vi "Update-motor-status.vi"(8 "error in (no error)":errorcluster, 11 "Object ref in":T1) -> (0 "error out":errorcluster, 3 "Object ref out":T1)   [LabVIEW 2013, in "PowderDeposition.lvlib" / "PD-Main.lvclass"]
uses:
  PD-Main.lvclass
  Object-reference.ctl
  PD-Main.lvclass/PD-Main.ctl
  Assembly/Motor-assembly.lvclass
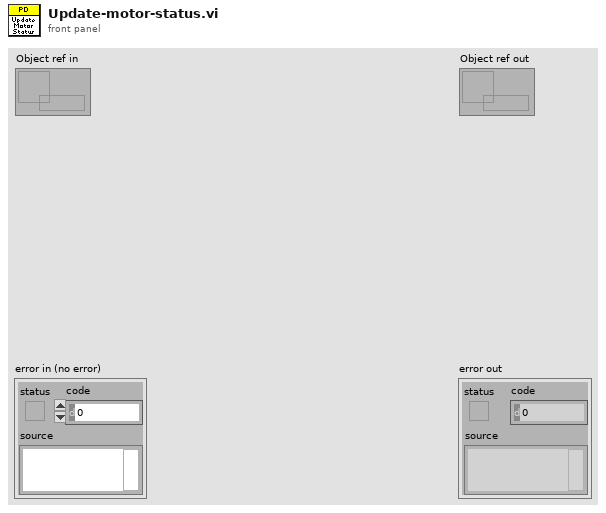
[diagram p1: front panel]
types:
  T1 = typedef "PowderDeposition.lvlib/PD-Main.lvclass/Object-reference.ctl" = refnum<data-value>
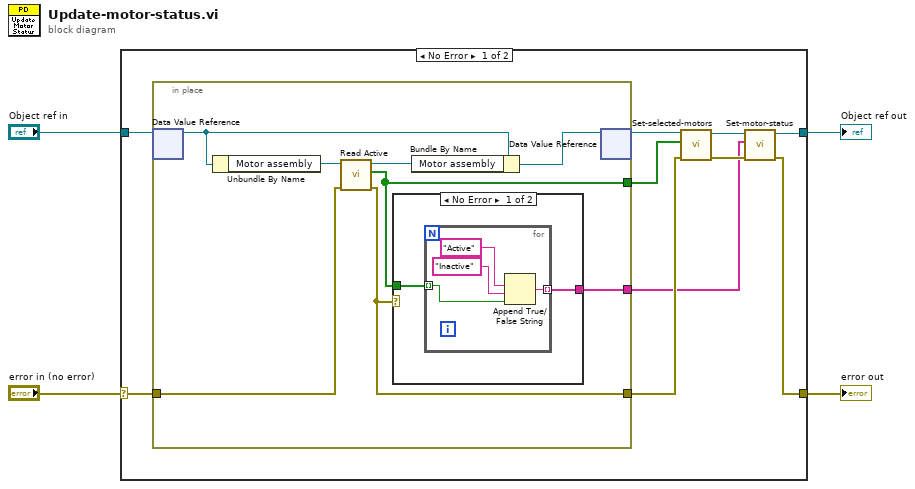
[diagram p0: block diagram]
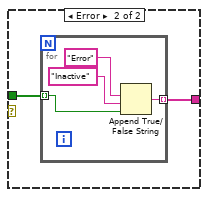
[diagram p2: hidden frame]
diagram:
  n1 = case shown="No Error" "error in (no error)" {
    selector: "error in (no error)" -> [w13 w36]
    tunnel: [w9 w36] -> w3
    tunnel: [w10 w35] -> w1
    tunnel: "Object ref in" -> [w14 w35]
    frame No Error {
      n2 = in-place {
        in-place-border: [w21] -> w8
        in-place-border: w13 -> [w20]
        in-place-border: [w16] -> w5
        in-place-border: [w15] -> w6
        n3 = in-place-dvr #1(w14) -> (w18:refnum<class "PD-Main.lvclass">)  [unwired: 1 out]
        n4 = Unbundle By Name(w18) -> ("Motor assembly"=w22:refnum<class "Motor-assembly.lvclass">)
        n5 = call-dynamic "Read Active.vi"("error in (no error)"=w20, "Available motors in"=w22) -> ("error out"=w21:errorcluster, "Active?"=w15:bool[], "Available motors out"=w19:refnum<class "Motor-assembly.lvclass">)  [unwired: 7 in]
        n6 = case shown="No Error" w21 {
          tunnel: w15 -> [w23 w30]
          tunnel: [w24 w29] -> w16
          frame No Error {
            n7 = for {
              tunnel: w23 -> [w28] mode=indexing
              tunnel: [w25] -> w24 mode=indexing
              n8 = Append True/False String(1:w28, 2:"Inactive" ("true string"), 3:"Active" ("true string")) -> (0:w25:string)  [unwired: 1 in]
            }
          }
          frame Error {
            n9 = for {
              tunnel: w30 -> [w34] mode=indexing
              tunnel: [w31] -> w29 mode=indexing
              n10 = Append True/False String(1:w34, 2:"Inactive" ("true string"), 3:"Error" ("true string")) -> (0:w31:string)  [unwired: 1 in]
            }
          }
        }
        n11 = Bundle By Name(cluster=w18, "Motor assembly"=w19) -> (w17:refnum<class "PD-Main.lvclass">)
        n12 = in-place-dvr #1(w17) -> (w12:T1)  [unwired: 1 out]
      }
      n13 = call "Set-selected-motors.vi"("error in (no error)"=w8, "Active?"=w6, "Object ref in"=w12) -> ("error out"=w7:errorcluster, "Object ref out"=w11:T1)  [unwired: 7 in]
      n14 = call "Set-motor-status.vi"("error in (no error)"=w7, "Status array"=w5, "Object ref in"=w11) -> ("error out"=w9:errorcluster, "Object ref out"=w10:T1)  [unwired: 7 in]
    }
    frame Error {
    }
  }
  "error out" <- w3
  "Object ref out" <- w1
